vi "Edit Substeps Analog Output.vi"(8 "error in":errorcluster, 9 "Station No":i32, 10 "AOWrite":T1, 11 "Sequence Context In":refnum<k7>) -> (0 "error out":errorcluster, 2 "AOWriteOut":T1, 3 "Report Text":string)   [LabVIEW 2023, in "LTT_TeststandSteptypes.lvlib"]
uses:
  LTT_TeststandSteptypes.lvlib
  HardwareAbstractionLayer_LVOOP/Database/SQL Public VI/Control/DB Options.ctl
  <vilib>/addons/TestStand/_TSUtility.llb/TestStand - Start Modal Dialog (Sequence Context).vi
  <vilib>/addons/TestStand/_TSUtility.llb/TestStand - End Modal Dialog (Sequence Context).vi
  HardwareAbstractionLayer_LVOOP/Database/Database.lvclass
panel:
  in  "Close":bool
  in  "OK":bool
  in  "Signal Name List":T2(array[cluster])
  in  "Signal Name":string(combo)
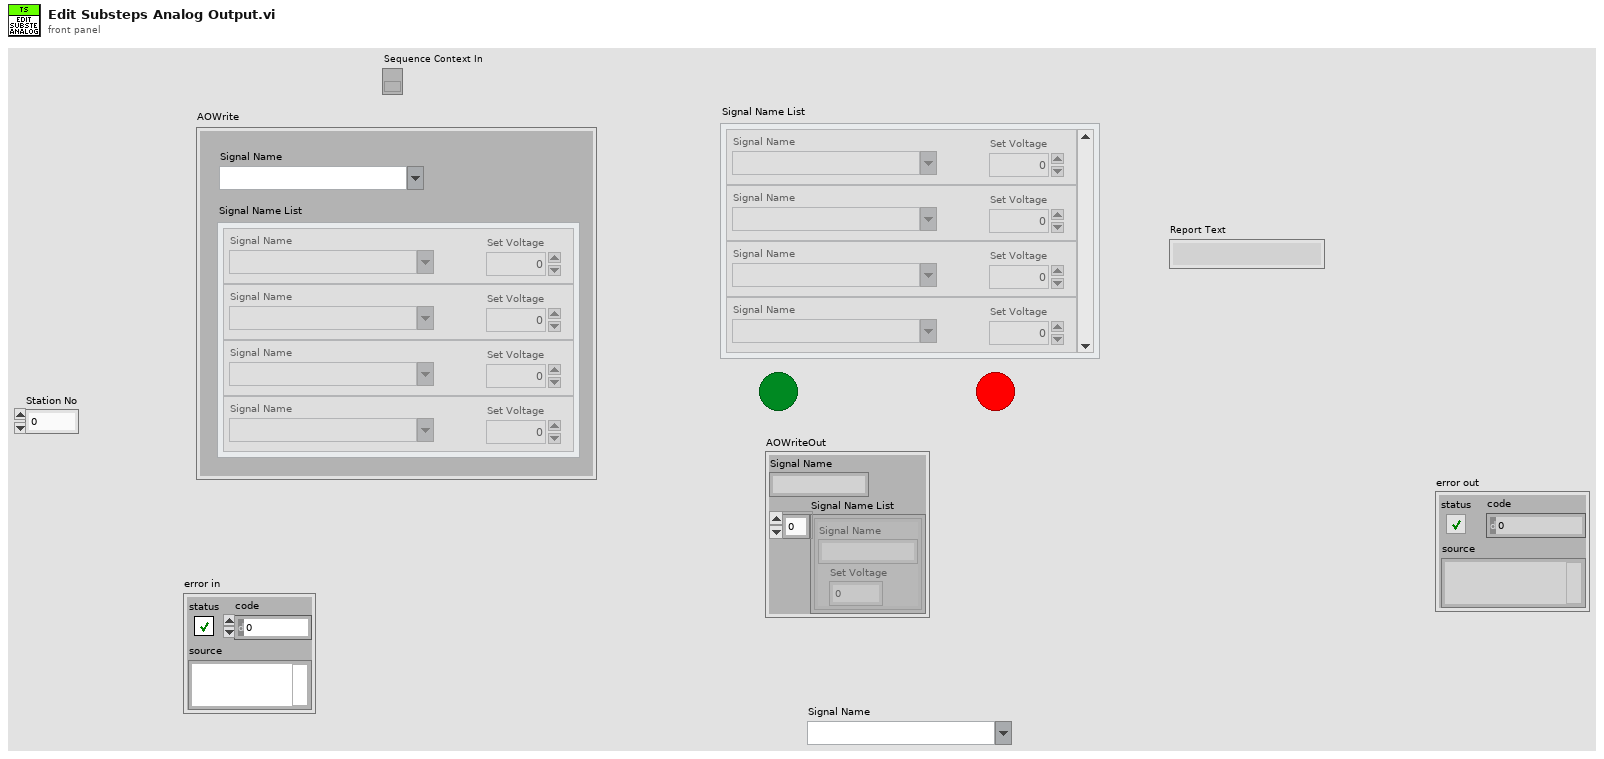
[diagram p1: front panel]
types:
  T1 = cluster{"Signal Name":string, "Signal Name List":cluster{"Signal Name":string, "Set Voltage":dbl}[]}
  T2 = cluster{"Signal Name":string, "Set Voltage":dbl}[]
  T3 = typedef "HardwareAbstractionLayer_LVOOP.lvlib/Database.lvclass/DB Options.ctl" = enum16{"Init", "Select Data", "Insert Data", "Update Data", "Delete Data", "Execute Query", "Create Schema", "Create Table", "List Tables", "List Columns", "Close"}
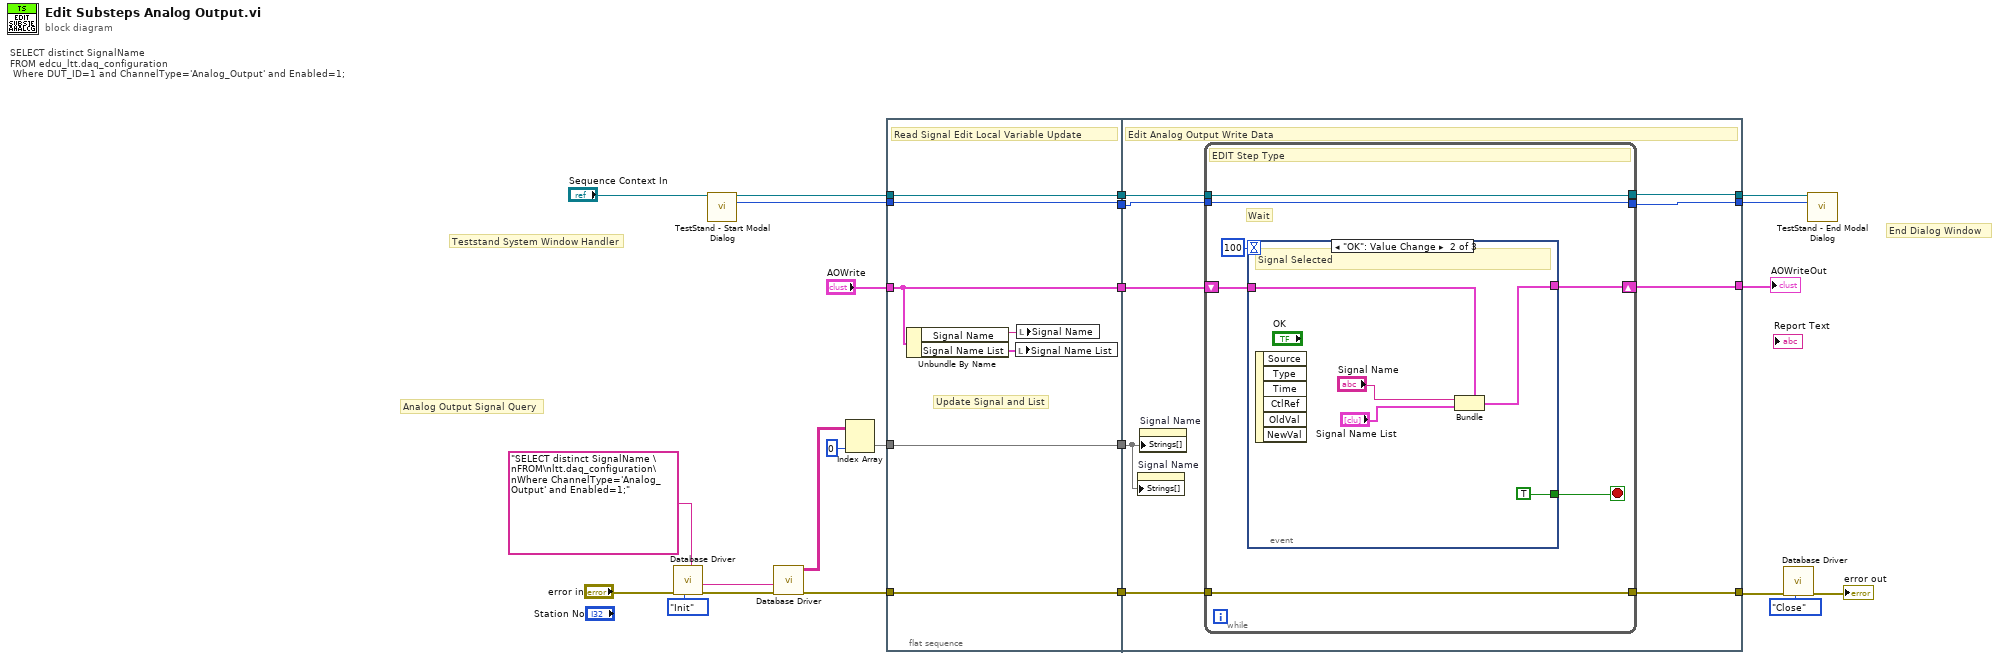
[diagram p0: block diagram]
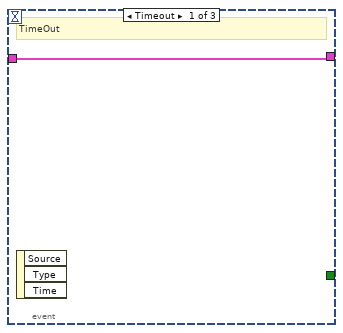
[diagram p2: hidden frame]
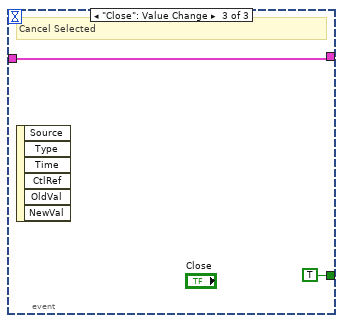
[diagram p3: hidden frame]
diagram:
  # "SELECT distinct SignalName \nFROM edcu_ltt.daq_configuration\n Where DUT_ID=1 and ChannelType='Analog_Output' and Enabled=1;"
  # "End Dialog Window"
  # "Teststand System Window Handler"
  # "Analog Output Signal Query"
  n1 = call "Database Driver.vi"("Options"=DB_Options."Init", "error in"="error in") -> ("error out"=w4:errorcluster)  [unwired: 6 in, 3 out]
  n2 = call-poly <vilib>:"TestStand - Start Modal Dialog.vi"("Sequence Context In"="Sequence Context In") -> ("Sequence Context Out"=w14:refnum<k7>, "Modal ID"=w13:i32)  [unwired: 10 in, 3 out]
  n3 = call "Database Driver.vi"("error in"=w4, "SQL query"="SELECT distinct SignalName \nFROM\nltt.daq_configuration\nWhere ChannelType='Analog_Output' and Enabled=1;") -> ("error out"=w10:errorcluster, "data"=w9:string[][])  [unwired: 6 in, 2 out]
  n4 = Index Array(array=w9, index (col)=0 ("disabled index (col)")) -> (element=w8:string[])  [unwired: 1 in]
  n5 = flat-sequence {
    tunnel: "AOWrite" -> [w28]
    tunnel: w10 -> [w30]
    tunnel: [w28] -> w22
    tunnel: [w30] -> w21
    tunnel: w14 -> [w29]
    tunnel: [w29] -> w19
    tunnel: w8 -> [w25]
    tunnel: [w25] -> w16
    tunnel: w13 -> [w24]
    tunnel: [w24] -> w12
    tunnel: w22 -> [w35]
    tunnel: w21 -> [w39]
    tunnel: [w38] -> w20
    tunnel: w19 -> [w37]
    tunnel: [w36] -> w18
    tunnel: [w31] -> w17
    tunnel: w16 -> [w34]
    tunnel: w12 -> [w33]
    tunnel: [w32] -> w11
    frame #0 {
      # "Update Signal and List"
      # "Read Signal Edit Local Variable Update"
      n6 = Unbundle By Name(w28) -> ("Signal Name"=w27:string, "Signal Name List"=w26:T2)
      n7 = local write "Signal Name List"(w26) -> ()
      n8 = local write "Signal Name"(w27) -> ()
    }
    frame #1 {
      # "Edit Analog Output Write Data"
      n9 = property on="Signal Name" class="CmbBox"("Strings[]"=w34) -> ()  [unwired: 2 in, 2 out]
      n10 = property on="Signal Name" class="CmbBox"("Strings[]"=w34) -> ()  [unwired: 2 in, 2 out]
      n11 = while {
        tunnel: w39 -> [w46]
        tunnel: [w46] -> w38
        tunnel: w37 -> [w45]
        tunnel: [w45] -> w36
        tunnel: w33 -> [w41]
        tunnel: [w41] -> w32
        shift-right: [w40] -> w31
        shift-left: w35 -> [w44]
        stop <- w42 stop-if-true
        # "Wait"
        # "EDIT Step Type"
        n12 = event shown="[1] \"OK\": Value Change" {
          selector: _ -> [_ _ _]
          dyn-events: _ -> [_ _ _]
          timeout: 100 -> [_ _ _]
          tunnel: w44 -> [w47 w51 w53]
          tunnel: [_ TRUE ("Stop") TRUE ("Stop")] -> w42
          tunnel: [w47 w48 w53] -> w40
          event Timeout {
            # "TimeOut"
            n13 = event-data() -> ()  [unwired: 1 in, 3 out]
          }
          event "OK": Value Change {
            # "Signal Selected"
            n14 = event-data() -> ()  [unwired: 1 in, 6 out]
            n15 = Bundle(cluster=w51, "Signal Name"="Signal Name", "Signal Name List"="Signal Name List") -> (w48:T1)
          }
          event "Close": Value Change {
            # "Cancel Selected"
            n16 = event-data() -> ()  [unwired: 1 in, 6 out]
          }
        }
      }
    }
  }
  n17 = call "Database Driver.vi"("Options"=DB_Options."Close", "error in"=w20) -> ("error out"=→"error out":errorcluster)  [unwired: 6 in, 3 out]
  n18 = call-poly <vilib>:"TestStand - End Modal Dialog.vi"("Sequence Context In"=w18, "Modal ID"=w11) -> ()  [unwired: 13 in, 1 out]
  "AOWriteOut" <- w17
